vi "calculate_filter_wash_speed.vi"(6 "timeout (25000ms)":i32=25000, 8 "error in (no error)":errorcluster, 10 "parameters":T1 {"C1" format="%#_20g"; "C2" format="%#_20g"; "C3" format="%#_21g"; "C4" format="%#_20g"}, 11 "daemon reference in":refnum<k5>) -> (0 "error out":errorcluster, 2 "response":string, 3 "daemon reference out":refnum<k5>, 5 "command out":string="random")   [LabVIEW 2017]
doc: "<b>Command: </b>\"template\"\n\n<b>Description: </b> This command does something.\n\n<b>Parameters: </b> None\n____________________________________________\nDIPC 692 Daemon API 10.0.0.1\nSam Tee - Dyson Technology Ltd\nCopyright (c) 2024, Dyson Technology Ltd"
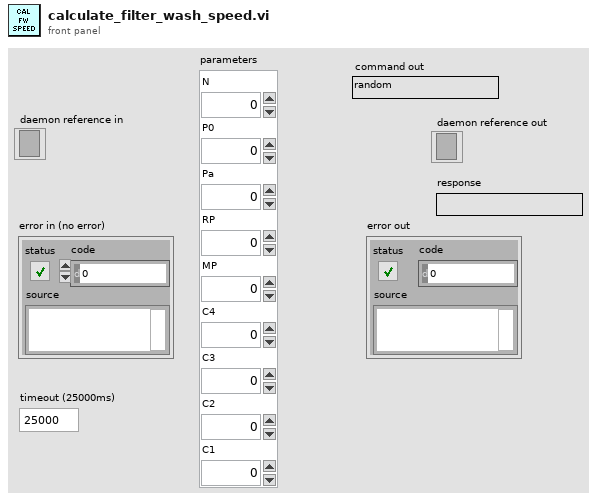
[diagram p1: front panel]
types:
  T1 = cluster{"N":dbl, "P0":dbl, "Pa":dbl, "RP":dbl, "MP":dbl, "C4":dbl, "C3":dbl, "C2":dbl, "C1":dbl}
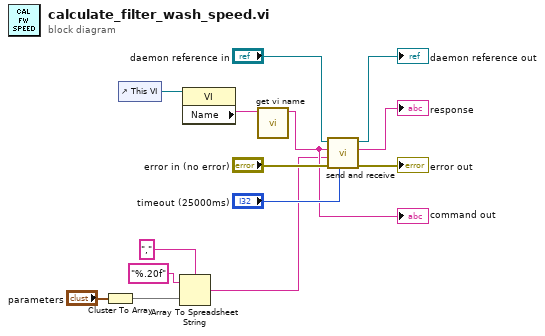
[diagram p0: block diagram]
diagram:
  n1 = Cluster To Array(cluster="parameters") -> (array=w4:dbl[])
  n2 = control-ref of="This VI"() -> (w8:refnum<vi>)
  n3 = Array To Spreadsheet String(delimiter (Tab)=",", array=w4, 3:"%.20f" ("format string")) -> (spreadsheet string=w1:string)
  n4 = property class="VI"(reference=w8) -> ("Name"=w7:string)  [unwired: 1 in, 2 out]
  n5 = call "get vi name.vi"("library.lvlib:name.vi"=w7) -> ("vi name"=w6:string)  [unwired: 10 in]
  "command out" <- w6
  n6 = call "send and receive.vi"("timeout (25000ms)"="timeout (25000ms)", "error in (no error)"="error in (no error)", "data"=w1, "command"=w6, "daemon reference in"="daemon reference in") -> ("error out"=→"error out":errorcluster, "response"=→"response":string, "daemon reference out"=→"daemon reference out":refnum<k5>)  [unwired: 4 in]
